vi "Set Callback On New Frame.vi"(10 "OnNewFrame":cluster{}, 11 "index":u16) -> (3 "function return":i32)   [LabVIEW 2025, in "ExtremelyEpicImagerIPC2.lvlib"]
doc: "IMAGERIPC_API HRESULT WINAPI SetCallback_OnAreasInit(WORD index, fpOnAreasInit OnAreasInit); IMAGERIPC_API HRESULT WINAPI SetCallback_OnNewFrame(WORD index, fpOnNewFrame OnNewFrame);"
uses:
  ExtremelyEpicImagerIPC2.lvlib
  ImagerIPC2.dll
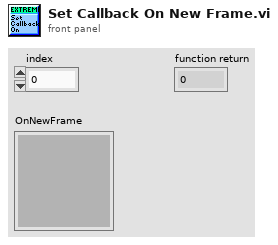
[diagram p1: front panel]
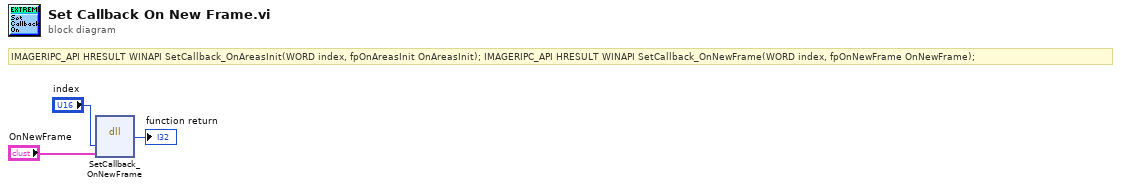
[diagram p0: block diagram]
diagram:
  # "IMAGERIPC_API HRESULT WINAPI SetCallback_OnAreasInit(WORD index, fpOnAreasInit OnAreasInit); IMAGERIPC_API HRESULT WINAPI SetCallback_OnNewFrame(WORD index, fpOnNewFrame OnNewFrame);"
  n1 = dll-call lib="C:/Users/mayhe/OneDrive/Documents/GitHub/In-situ-monitoring-of-powder-bed-fusion-additive-manufacturing/system_development/Orichalcum/v0.2/Software_design/thermal-camera/VI/Connect SDK/ImagerIPC2.*" fn="SetCallback_OnNewFrame"("index"="index", "OnNewFrame"="OnNewFrame") -> (→"function return":i32)  [unwired: 5 in, 2 out]
